vi "SaveInterfSetup.vi"(8 "error in (no error)":errorcluster caption="entrée d'erreur (pas d'erreur)", 10 "Allow Save":bool, 11 "Interface en entrée":refnum<class "Interface.lvclass"> caption="DNL_LabVIEW Object in") -> (0 "error out":errorcluster caption="sortie d'erreur", 2 "SavePath":path, 3 "Interface en sortie":refnum<class "Interface.lvclass"> caption="DNL_LabVIEW Object out")   [LabVIEW 2010, in "Interface.lvclass"]
uses:
  Interface.lvclass
  SetInitPar.ctl
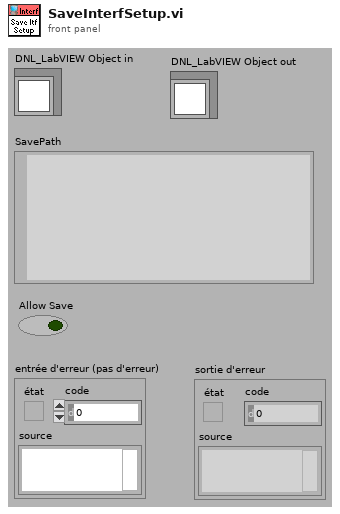
[diagram p1: front panel]
types:
  T1 = typedef "SetInitPar.ctl" = enum16{"All", "GraphConfig", "ScanFormats", "ScanPref", "LogPref", "BasePath", "Experiment"}
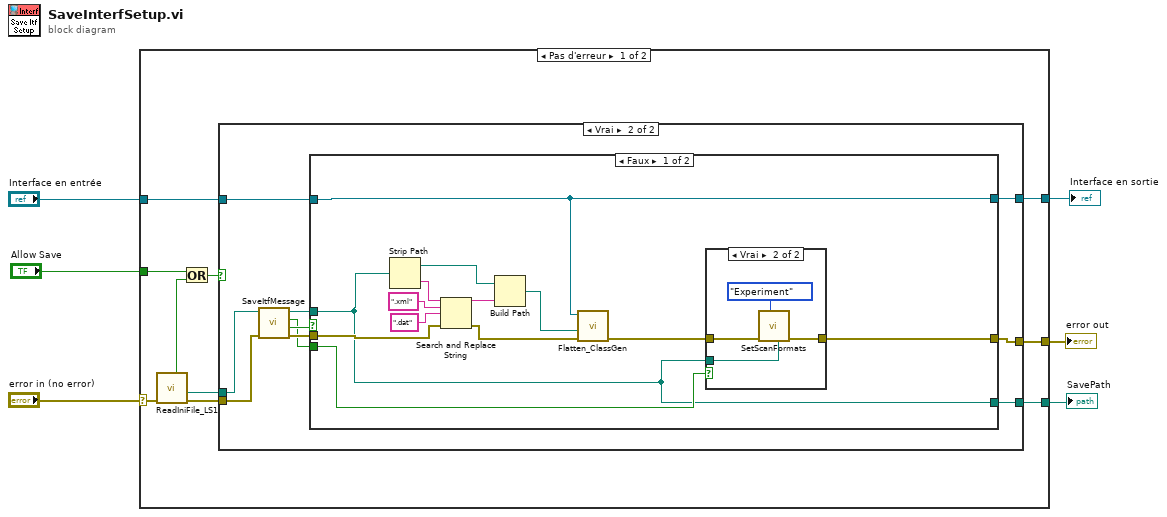
[diagram p0: block diagram]
diagram:
  n1 = case shown="Pas d'erreur" "error in (no error)" {
    selector: "error in (no error)" -> [w14 w50]
    tunnel: [w15 w50] -> w5
    tunnel: [w12 w49] -> w3
    tunnel: "Interface en entrée" -> [w16 w49]
    tunnel: [w10 _] -> w2
    tunnel: "Allow Save" -> [w9 _]
    frame No Error {
      n2 = call "ReadIniFile_LS1.vi"("Error in"=w14) -> ("Error out"=w11:errorcluster, "Experiment"=w13:path, "AllowSave"=w8:bool)  [unwired: 5 in, 3 out]
      n3 = Or(x=w9, y=w8) -> (x .or. y?=w7:bool)
      n4 = case shown="Vrai" w7 {
        tunnel: w16 -> [w18 w27]
        tunnel: [w17 w28] -> w15
        tunnel: w13 -> [_ w26]
        tunnel: [w18 w20] -> w12
        tunnel: w11 -> [w17 w25]
        tunnel: [_ w19] -> w10
        frame False {
        }
        frame True {
          n5 = call "SaveItfMessage.vi"("error in (no error)"=w25, "cheminIn"=w26) -> ("error out"=w24:errorcluster, "Cancel Out"=w22:bool, "StartITF Out"=w21:bool, "CheminOut"=w23:path)  [unwired: 6 in]
          n6 = case shown="Faux" w22 {
            tunnel: [w35 w47] -> w28
            tunnel: w27 -> [w30 w48]
            tunnel: w24 -> [w37 w47]
            tunnel: w23 -> [w33 _]
            tunnel: w21 -> [w34 _]
            tunnel: [w30 w48] -> w20
            tunnel: [w33 _] -> w19
            frame False {
              n7 = Strip Path(path=w33) -> (stripped path=w40:path, name=w41:string)
              n8 = Search and Replace String(input string=w41, search string=".xml" ("chaîne recherchée"), replace string=".dat" ("chaîne de remplacement (\"\")"), error in=w37) -> (result string=w36:string, error out=w31:errorcluster)  [unwired: 4 in, 2 out]
              n9 = Build Path(base path=w40, name or relative path=w36) -> (appended path=w29:path)
              n10 = call <userlib>:"Flatten_ClassGen.vi"("error in (no error)"=w31, "XML File Path"=w29, "Objet LabVIEW"=w30) -> ("error out"=w32:errorcluster)  [unwired: 6 in, 2 out]
              n11 = case shown="Vrai" w34 {
                tunnel: w33 -> [_ w45]
                tunnel: w32 -> [w42 w44]
                tunnel: [w42 w43] -> w35
                frame False {
                }
                frame True {
                  n12 = call "SetScanFormats.vi"("Experiment"=w45, "Énum"=SetInitPar."Experiment", "ErrorIn(No Error)"=w44) -> ("sortie d'erreur"=w43:errorcluster)  [unwired: 8 in]
                }
              }
            }
            frame True {
            }
          }
        }
      }
    }
    frame Error {
    }
  }
  "error out" <- w5
  "Interface en sortie" <- w3
  "SavePath" <- w2
